vi "Read_CANUSB.vi"(5 "VISA  in":refnum<visa-resource-name>, 6 "byte count":u32) -> (0 "VISA  out":refnum<visa-resource-name>, 1 "Status":bool, 2 "TPCANMsg out":T1 {"ID" format="%x"; "MSGTYPE" items=["STATUS"=128, "EXTENDED"=2, "RTR"=1, "DATA MSG"=0]; "aDATA" format="%x"}, 3 "error out 5":errorcluster, 4 "read buffer":string)   [LabVIEW 2017]
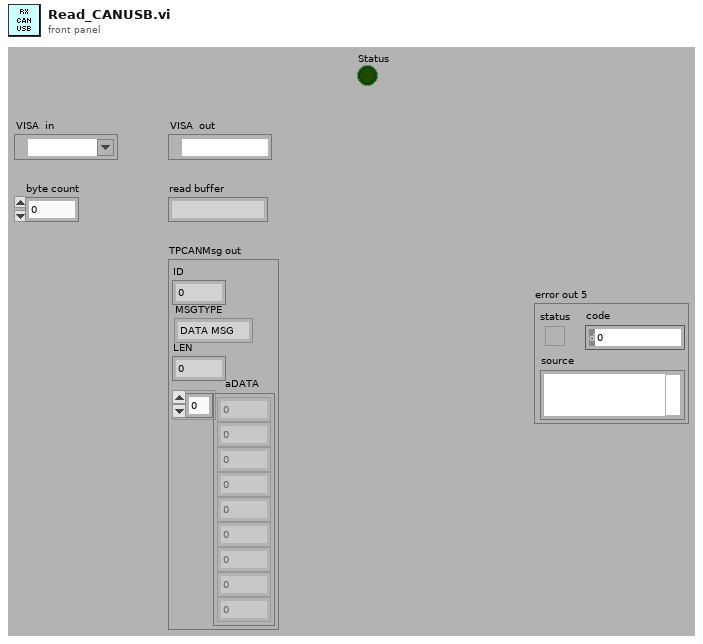
[diagram p1: front panel]
types:
  T1 = cluster{"ID":u32, "MSGTYPE":u8, "LEN":u8, "aDATA":u8[]}
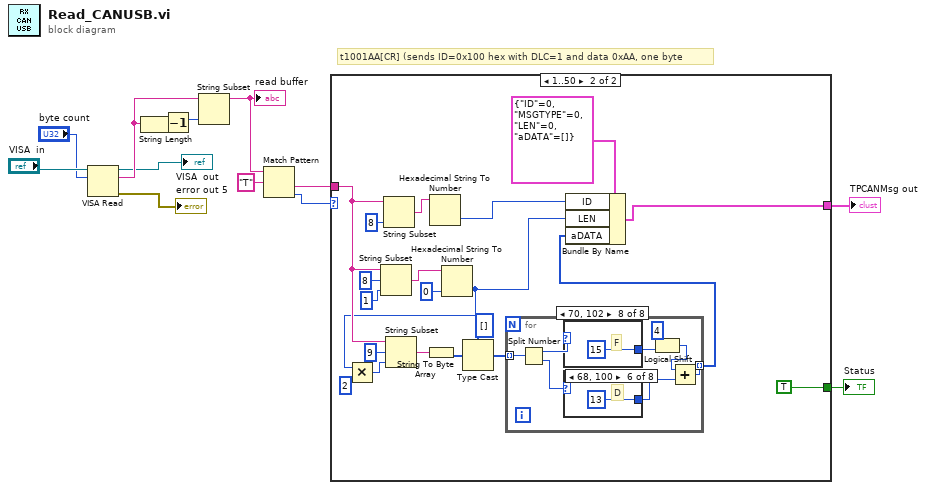
[diagram p0: block diagram]
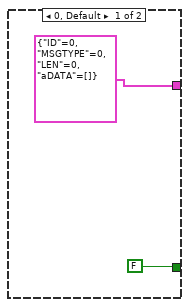
[diagram p2: hidden frame]
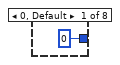
[diagram p3: hidden frame]
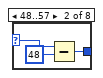
[diagram p4: hidden frame]
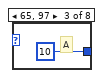
[diagram p5: hidden frame]
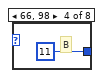
[diagram p6: hidden frame]
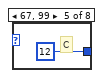
[diagram p7: hidden frame]
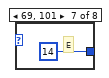
[diagram p8: hidden frame]
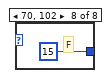
[diagram p9: hidden frame]
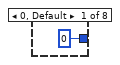
[diagram p10: hidden frame]
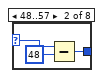
[diagram p11: hidden frame]
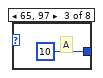
[diagram p12: hidden frame]
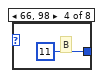
[diagram p13: hidden frame]
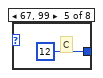
[diagram p14: hidden frame]
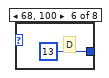
[diagram p15: hidden frame]
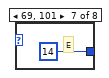
[diagram p16: hidden frame]
diagram:
  # "t1001AA[CR] (sends ID=0x100 hex with DLC=1 and data 0xAA, one byte"
  n1 = VISA Read(VISA resource name="VISA  in", byte count="byte count") -> (VISA resource name out=→"VISA  out":refnum<visa-resource-name>, read buffer=w9:string, error out=→"error out 5":errorcluster)  [unwired: 1 in, 1 out]
  n2 = String Length(string=w9) -> (length=w7:i32)
  n3 = Decrement(x=w7) -> (x-1=w8:i32)
  n4 = String Subset(string=w9, length (rest)=w8) -> (substring=w10:string)  [unwired: 1 in]
  "read buffer" <- w10
  n5 = Match Pattern(string=w10, regular expression="T") -> (after substring=w12:string, offset past match=w2:i32)  [unwired: 1 in, 2 out]
  n6 = case shown="1..50" w2 {
    tunnel: w12 -> [_ w29]
    tunnel: [T1 {"ID"=0, "MSGTYPE"=0, "LEN"=0, "aDATA"=[]} ("TPCANMsg 3") w20] -> w3
    tunnel: [FALSE TRUE] -> w1
    frame 0, Default {
    }
    frame 1..50 {
      n7 = String Subset(string=w29, offset (0)=8, length (rest)=1 ("length (rest)")) -> (substring=w27:string)
      n8 = String Subset(string=w29, length (rest)=8 ("length (rest)")) -> (substring=w22:string)  [unwired: 1 in]
      n9 = Hexadecimal String To Number(string=w22) -> (number=w24:u32)  [unwired: 2 in, 1 out]
      n10 = Hexadecimal String To Number(string=w27, default (0uL)=u8 0 ("default (0 U32)")) -> (number=w17:u8)  [unwired: 1 in, 1 out]
      n11 = Multiply(x=w17, y=u8 2) -> (x*y=w18:u8)
      n12 = String Subset(string=w29, offset (0)=9, length (rest)=w18) -> (substring=w31:string)
      n13 = String To Byte Array(string=w31) -> (unsigned byte array=w33:u8[])
      n14 = Type Cast(type=u16[] [], x=w33) -> (*(type *) &x=w34:u16[])
      n15 = for {
        tunnel: w34 -> [w43] mode=indexing
        tunnel: [w36] -> w35 mode=indexing
        n16 = Split Number(x=w43) -> (hi(x)=w42:u8, lo(x)=w41:u8)
        n17 = case shown="70, 102" w42 {
          selector: w42 -> [_ w57 _ _ _ _ _ _]
          tunnel: [u8 0 ("y") w55 u8 10 ("y") u8 11 ("y") u8 12 ("y") u8 13 ("y") u8 14 ("y") u8 15 ("y")] -> w40
          frame 0, Default {
          }
          frame 48..57 {
            n18 = Subtract(x=w57, y=u8 48) -> (x-y=w55:u8)
          }
          frame 65, 97 {
            # "A"
          }
          frame 66, 98 {
            # "B"
          }
          frame 67, 99 {
            # "C"
          }
          frame 68, 100 {
            # "D"
          }
          frame 69, 101 {
            # "E"
          }
          frame 70, 102 {
            # "F"
          }
        }
        n19 = case shown="68, 100" w41 {
          selector: w41 -> [_ w47 _ _ _ _ _ _]
          tunnel: [u8 0 ("y") w45 u8 10 ("y") u8 11 ("y") u8 12 ("y") u8 13 ("y") u8 14 ("y") u8 15 ("y")] -> w37
          frame 0, Default {
          }
          frame 48..57 {
            n20 = Subtract(x=w47, y=u8 48) -> (x-y=w45:u8)
          }
          frame 65, 97 {
            # "A"
          }
          frame 66, 98 {
            # "B"
          }
          frame 67, 99 {
            # "C"
          }
          frame 68, 100 {
            # "D"
          }
          frame 69, 101 {
            # "E"
          }
          frame 70, 102 {
            # "F"
          }
        }
        n21 = Logical Shift(y=i8 4, x=w40) -> (x << y=w38:u8)
        n22 = Add(x=w38, y=w37) -> (x+y=w36:u8)
      }
      n23 = Bundle By Name(cluster=T1 {"ID"=0, "MSGTYPE"=0, "LEN"=0, "aDATA"=[]} ("TPCANMsg 3"), "ID"=w24, "LEN"=w17, "aDATA"=w35) -> (w20:T1)
    }
  }
  "TPCANMsg out" <- w3
  "Status" <- w1
